vi "Init.vi"(8 "error in (no error)":errorcluster, 11 "reference in":refnum<class "DMM_Keysight_34980A.lvclass">) -> (0 "error out":errorcluster, 3 "reference out":refnum<class "DMM_Keysight_34980A.lvclass">)   [LabVIEW 2022 SP3, in "DMM_Keysight_34980A.lvlib" / "DMM_Keysight_34980A.lvclass"]
uses:
  DMM_Keysight_34980A.lvclass
  Components/ViPER.lvlibp/ViPER.lvclass
  C:/Projects/Medulla/ViPER/Examples/Flux_Capacitor_Tester/Components/ViPER.lvlibp/ViPER.lvclass
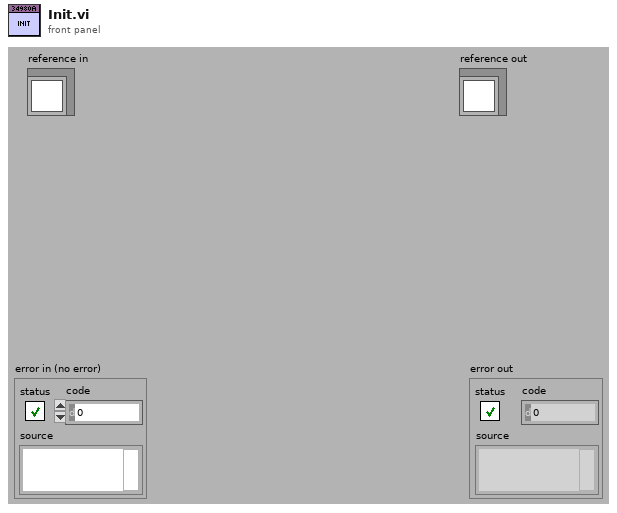
[diagram p1: front panel]
types:
  T1 = enum16{"4 1/2", "5 1/2", "6 1/2", "Least", "Highest", "Default"}
  T2 = typedef "DMM_Keysight_34980A.lvlib/DMM_Keysight_34980A.lvclass/ObjectAttributes.ctl" = cluster{"Config":T3, "VISA ref":refnum<visa-resource-name>, "Meas":dbl, "Range DCV":enum16{"100 mV", "1 V", "10 V", "100 V", "300 V", "Auto", "Minimum", "Maximum"}, "Range ACV":enum16{"100 mV", "1 V", "10 V", "100 V", "300 V", "Auto", "Minimum", "Maximum", "Default"}, "Range Ohms":enum16{"100 Ohm", "1 kOhm", "10 kOhm", "100 kOhm", "1 MOhm", "10 MOhm", "100 MOhm", "Auto", "Minimum", "Maximum"}, "Range VFreq":enum16{"100 mV", "1 V", "10 V", "100 V", "300 V", "Auto", "Minimum", "Maximum"}, " Range ACA":enum16{"10 mA", "100 mA", "1 A", "Auto", "Minimum", "Maximum"}, " Range DCA":enum16{"10 mA", "100 mA", "1 A", "Auto", "Minimum", "Maximum"}, "Mode":T4, "Resolution":enum16{"4 1/2", "5 1/2", "6 1/2", "Least", "Highest", "Default"}, "Bandwidth":enum16{"3 Hz", "20 Hz", "200 Hz", "Minimum", "Maximum"}, "Low Frequency":enum16{"3 Hz", "20 Hz", "200 Hz", "Minimum", "Maximum"}, "Aperture":enum16{"10 ms", "100 ms", "1 sec", "Minimum", "Maximum"}, "Measurement":dbl[], "Time":dbl[], "Samples":u32, "dt":dbl, "Timeout":dbl}
  T3 = typedef "DMM_Keysight_34980A.lvlib/DMM_Keysight_34980A.lvclass/Config.ctl" = cluster{"VISA":refnum<visa-resource-name>}
  T4 = typedef "DMM_Keysight_34980A.lvlib/DMM_Keysight_34980A.lvclass/Mode.ctl" = enum16{"DCV", "ACV", "2W Ohms", "4W Ohms", "Frequency", "DCA", "ACA"}
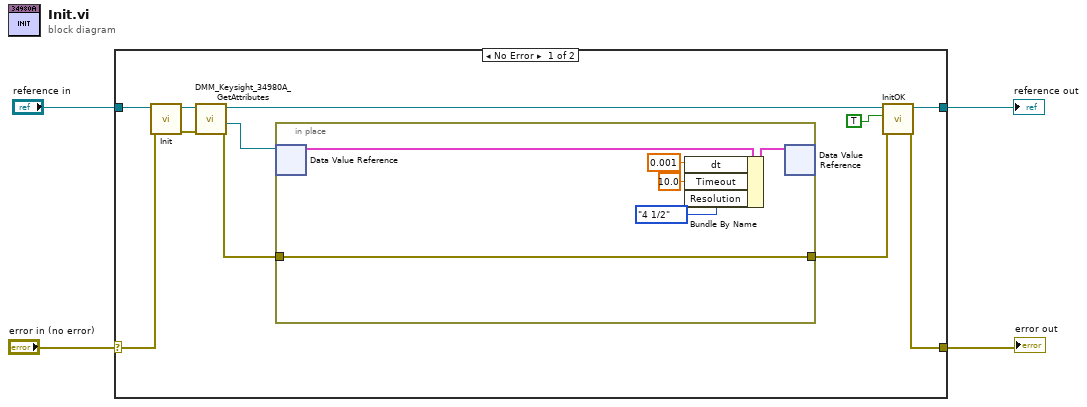
[diagram p0: block diagram]
diagram:
  n1 = case shown="No Error" "error in (no error)" {
    selector: "error in (no error)" -> [w14 w23]
    tunnel: [w5 w23] -> w3
    tunnel: [w8 w22] -> w1
    tunnel: "reference in" -> [w15 w22]
    frame No Error {
      n2 = call-parent "Init.vi"("error in (no error)"=w14, "reference in"=w15) -> ("error out"=w12:errorcluster, "reference out"=w13:refnum<class "DMM_Keysight_34980A.lvclass">)  [unwired: 8 in]
      n3 = call "DMM_Keysight_34980A_GetAttributes.vi"("error in (no error)"=w12, "reference in"=w13) -> ("error out"=w10:errorcluster, "DataRef"=w11:refnum<data-value>, "reference out"=w9:refnum<class "DMM_Keysight_34980A.lvclass">)  [unwired: 6 in, 1 out]
      n4 = in-place {
        in-place-border: w10 -> [w16]
        in-place-border: [w16] -> w6
        n5 = in-place-dvr #1(w11) -> (w21:T2)  [unwired: 1 out]
        n6 = Bundle By Name(cluster=w21, "dt"=0.001, "Timeout"=10.0, "Resolution"=T1."4 1/2") -> (w20:T2)
        n7 = in-place-dvr #1(w20) -> ()  [unwired: 2 out]
      }
      n8 = call "InitOK.vi"("error in (no error)"=w6, "Init OK?"=TRUE, "reference in"=w9) -> ("error out"=w5:errorcluster, "reference out"=w8:refnum<class "DMM_Keysight_34980A.lvclass">)  [unwired: 7 in]
    }
    frame Error {
    }
  }
  "error out" <- w3
  "reference out" <- w1
